vi "Set Window Color to Transparent.vi"(5 "error in (no error)":errorcluster) -> (0 "error out":errorcluster)   [LabVIEW 2020]
uses:
  user32.dll
panel:
  # "Input"
  # "Output"
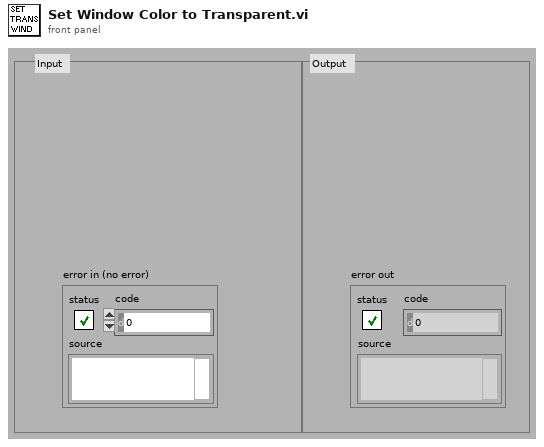
[diagram p1: front panel]
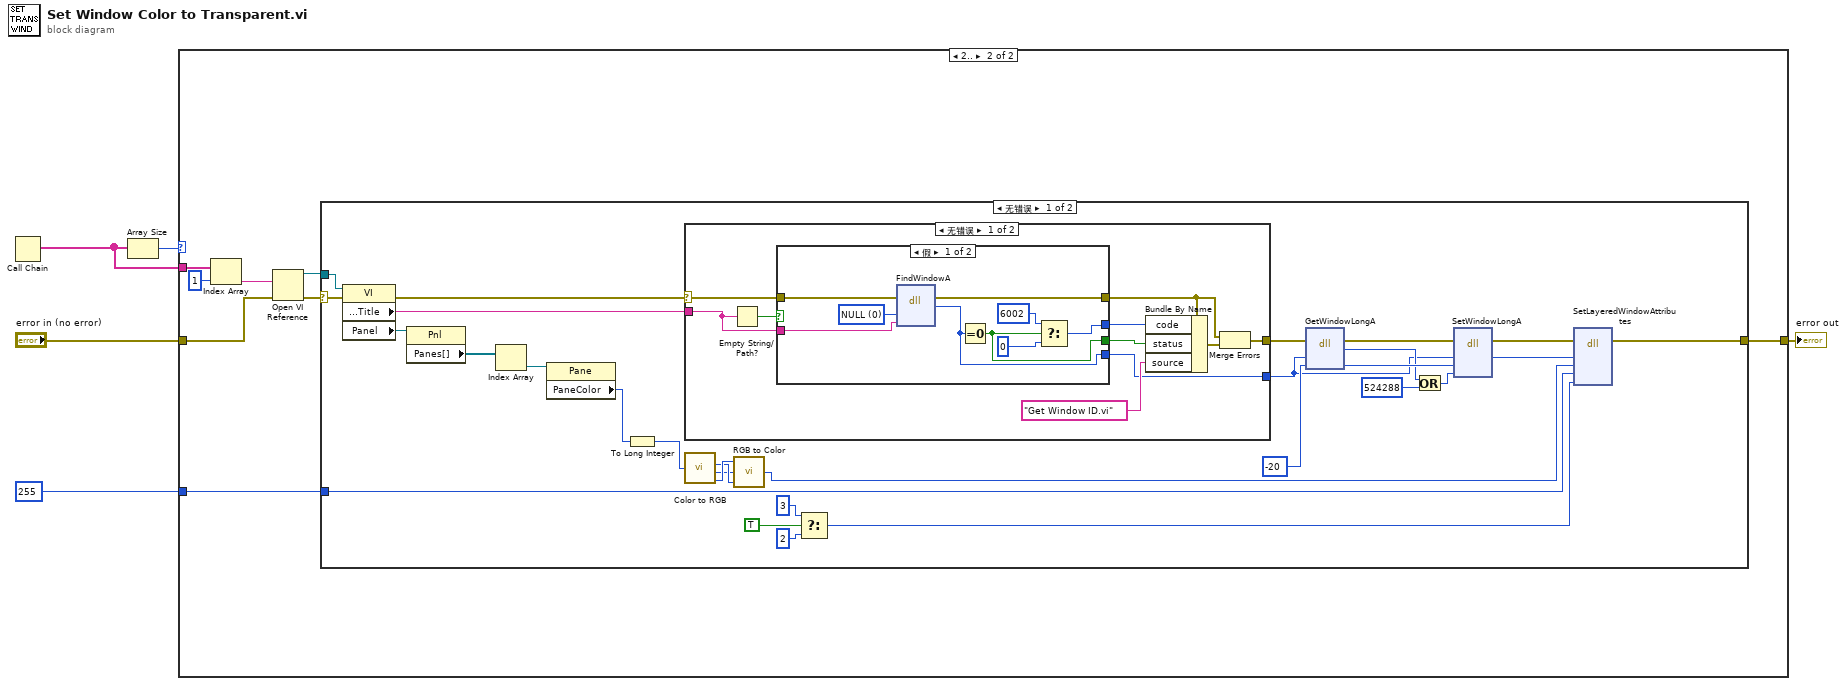
[diagram p0: block diagram]
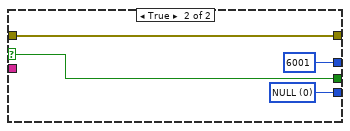
[diagram p3: hidden frame]
diagram:
  n1 = Call Chain() -> (call chain=w4:string[])
  n2 = Array Size(array=w4) -> (size(s)=w3:i32)
  n3 = case shown="2.." w3 {
    tunnel: [w6 w14] -> w5
    tunnel: w4 -> [_ w13]
    tunnel: "error in (no error)" -> [w6 w9]
    tunnel: u8 255 ("Factor") -> [_ w7]
    frame 0, Default {
    }
    frame 2.. {
      n4 = Index Array(array=w13, index=1 ("索引")) -> (element=w11:string)
      n5 = Open VI Reference(vi path=w11, error in (no error)=w9) -> (vi reference=w10:refnum<vi>, error out=w8:errorcluster)  [unwired: 4 in]
      n6 = case shown="无错误" w8 {
        selector: w8 -> [w21 w68]
        tunnel: w10 -> [w31 _]
        tunnel: w7 -> [w24 _]
        tunnel: [w22 w68] -> w14
        frame No Error {
          n7 = property class="VI"(reference=w31, error in=w21) -> (error out=w32:errorcluster, "Front Panel.Title"=w30:string, "Panel"=w18:refnum<vi>)  [unwired: 1 out]
          n8 = property class="Pnl"(reference=w18) -> ("Panes[]"=w17:refnum<vi>[])  [unwired: 1 in, 2 out]
          n9 = Index Array(array=w17) -> (element=w16:refnum<vi>)  [unwired: 1 in]
          n10 = property class="Pane"(reference=w16) -> ("PaneColor"=w15:u32)  [unwired: 1 in, 2 out]
          n11 = To Long Integer(number=w15) -> (32bit integer=w40:i32)
          n12 = case shown="无错误" w32 {
            selector: w32 -> [w45 w67]
            tunnel: [w47 w67] -> w33
            tunnel: [w50 _] -> w20
            tunnel: w30 -> [w46 _]
            frame No Error {
              n13 = Empty String/Path?(string/path=w46) -> (empty?=w49:bool)
              n14 = case shown="假" w49 {
                selector: w49 -> [_ w64]
                tunnel: [w62 w65] -> w50
                tunnel: [w61 w64] -> w52
                tunnel: [w60 6001] -> w53
                tunnel: w46 -> [w56 _]
                tunnel: w45 -> [w55 w63]
                tunnel: [w54 w63] -> w44
                frame False {
                  w57 = 0 items=["NULL"]
                  n15 = dll-call lib="user32.dll" fn="FindWindowA" label="FindWindow"(error in=w55, "lpszClassName"=w57, "lpszWindowName"=w56) -> (error out=w54:errorcluster, "hWnd"=w62:u32)  [unwired: 4 in, 1 out]
                  n16 = Equal To 0?(x=w62) -> (x = 0?=w61:bool)
                  n17 = Select(t=6002, s=w61, f=0) -> (s? t:f=w60:i32)
                }
                frame True {
                  w65 = u16 0 items=["NULL"]
                }
              }
              n18 = Bundle By Name(cluster=w44, "code"=w53, "status"=w52, "source"="Get Window ID.vi") -> (w48:errorcluster)
              n19 = Merge Errors(w44, w48) -> (w47:errorcluster)
            }
            frame Error {
            }
          }
          n20 = call <vilib>:"Color to RGB.vi"("Color"=w40) -> ("R"=w38:u8, "G"=w37:u8, "B"=w39:u8)  [unwired: 1 out]
          n21 = call <vilib>:"RGB to Color.vi"("B"=w38, "G"=w37, "R"=w39) -> ("Color"=w41:u32)
          n22 = Select(t=3, s=TRUE, f=2) -> (s? t:f=w34:i32)
          n23 = dll-call lib="user32.dll" fn="GetWindowLongA" label="getWindowLong"(error in=w33, "handle"=w20, "nIndex"=-20) -> (error out=w26:errorcluster, w28:i32, "nIndex"=w43:i32)  [unwired: 3 in, 1 out]
          n24 = Or(x=w28, y=524288) -> (x .or. y?=w25:i32)
          n25 = dll-call lib="user32.dll" fn="SetWindowLongA" label="SetWindowLong"(error in=w26, "handle"=w20, "nIndex"=w43, "dwNewLong"=w25) -> (error out=w27:errorcluster, "handle"=w23:i32)  [unwired: 4 in, 2 out]
          n26 = dll-call lib="user32.dll" fn="SetLayeredWindowAttributes" label="SetLayerdWindowAttributs"(error in=w27, "handle"=w23, "crkey"=w41, "bAlpha"=w24, "dwFlags"=w34) -> (error out=w22:errorcluster)  [unwired: 5 in, 3 out]
        }
        frame Error {
        }
      }
    }
  }
  "error out" <- w5
